vi "getStopMechanism.vi"(8 "error in (no error)":errorcluster, 11 "ExampleTask_StopNotifier in":refnum<class "ExampleTask_BoolUserEventStop.lvclass">) -> (0 "error out":errorcluster, 2 "stopMechanism":refnum<class "ITaskStopMechanism.lvclass">, 3 "ExampleTask_StopNotifier out":refnum<class "ExampleTask_BoolUserEventStop.lvclass">)   [LabVIEW 2023, in "ExampleTask_BoolUserEventStop.lvclass"]
doc: "Returns the stop mechanism type used by the task."
uses:
  ExampleTask_BoolUserEventStop.lvclass
  ITaskStopMechanism/ITaskStopMechanism.lvclass
  BoolUserEventStopMech/BoolUserEventStopMechanism.lvclass
  ExampleTask_BoolUserEventStop.lvclass/ExampleTask_BoolUserEventStop.ctl
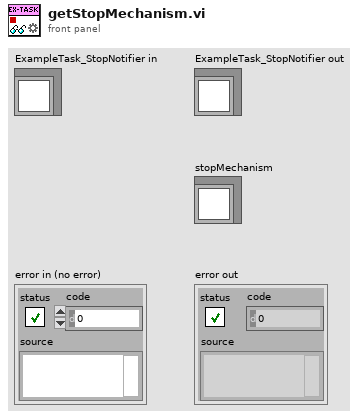
[diagram p1: front panel]
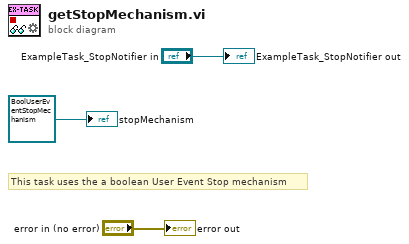
[diagram p0: block diagram]
diagram:
  # "This task uses the a boolean User Event Stop mechanism"
  "error out" <- "error in (no error)"
  "ExampleTask_StopNotifier out" <- "ExampleTask_StopNotifier in"
  "stopMechanism" <- refnum<class "BoolUserEventStopMechanism.lvclass"> refnum ("TLC_Daemon.lvlib:BoolUserEventStopMechanism.lvclass")
